vi "GUI_Plasma2_MedJet.vi"() -> ()   [LabVIEW 2013]
uses:
  Shared/GUI_Template/GUI_master/tcp_new_data_event.ctl
  Shared/GUI_Template/GUI_master/tcp new data cluster.ctl
  Control 1.ctl
panel:
  in  "PressureSetPoint.device 1::1":dbl=0.001 caption="Alicat HP Set" min=0.0 max=20.0 format="%_4f"
  in  "PressureSetPoint.device 2::1":dbl=0.001 caption="Alicat LP Set" min=0.0 max=20.0 format="%_4f"
  in  "GUIdevice 1":T1="PL2-PresCtl" caption="PL2-PresCtrl"
  in  "stop":bool
  in  "All Off":bool
  in  "PressureReading.device 1::1":dbl=0.001 caption="Alicat HP Read" min=-10.0 max=20.0 format="%_4f"
  in  "PressureReading.device 2::1":dbl=0.001 caption="Alicat LP Read" min=-10.0 max=20.0 format="%_4f"
  in  "High Valve":bool
  in  "Low Valve":bool
  in  "LN Set Pressure":dbl
  in  "HN Set Pressure":dbl
  out "tcp data event":T2
  out "error IO 2":errorcluster
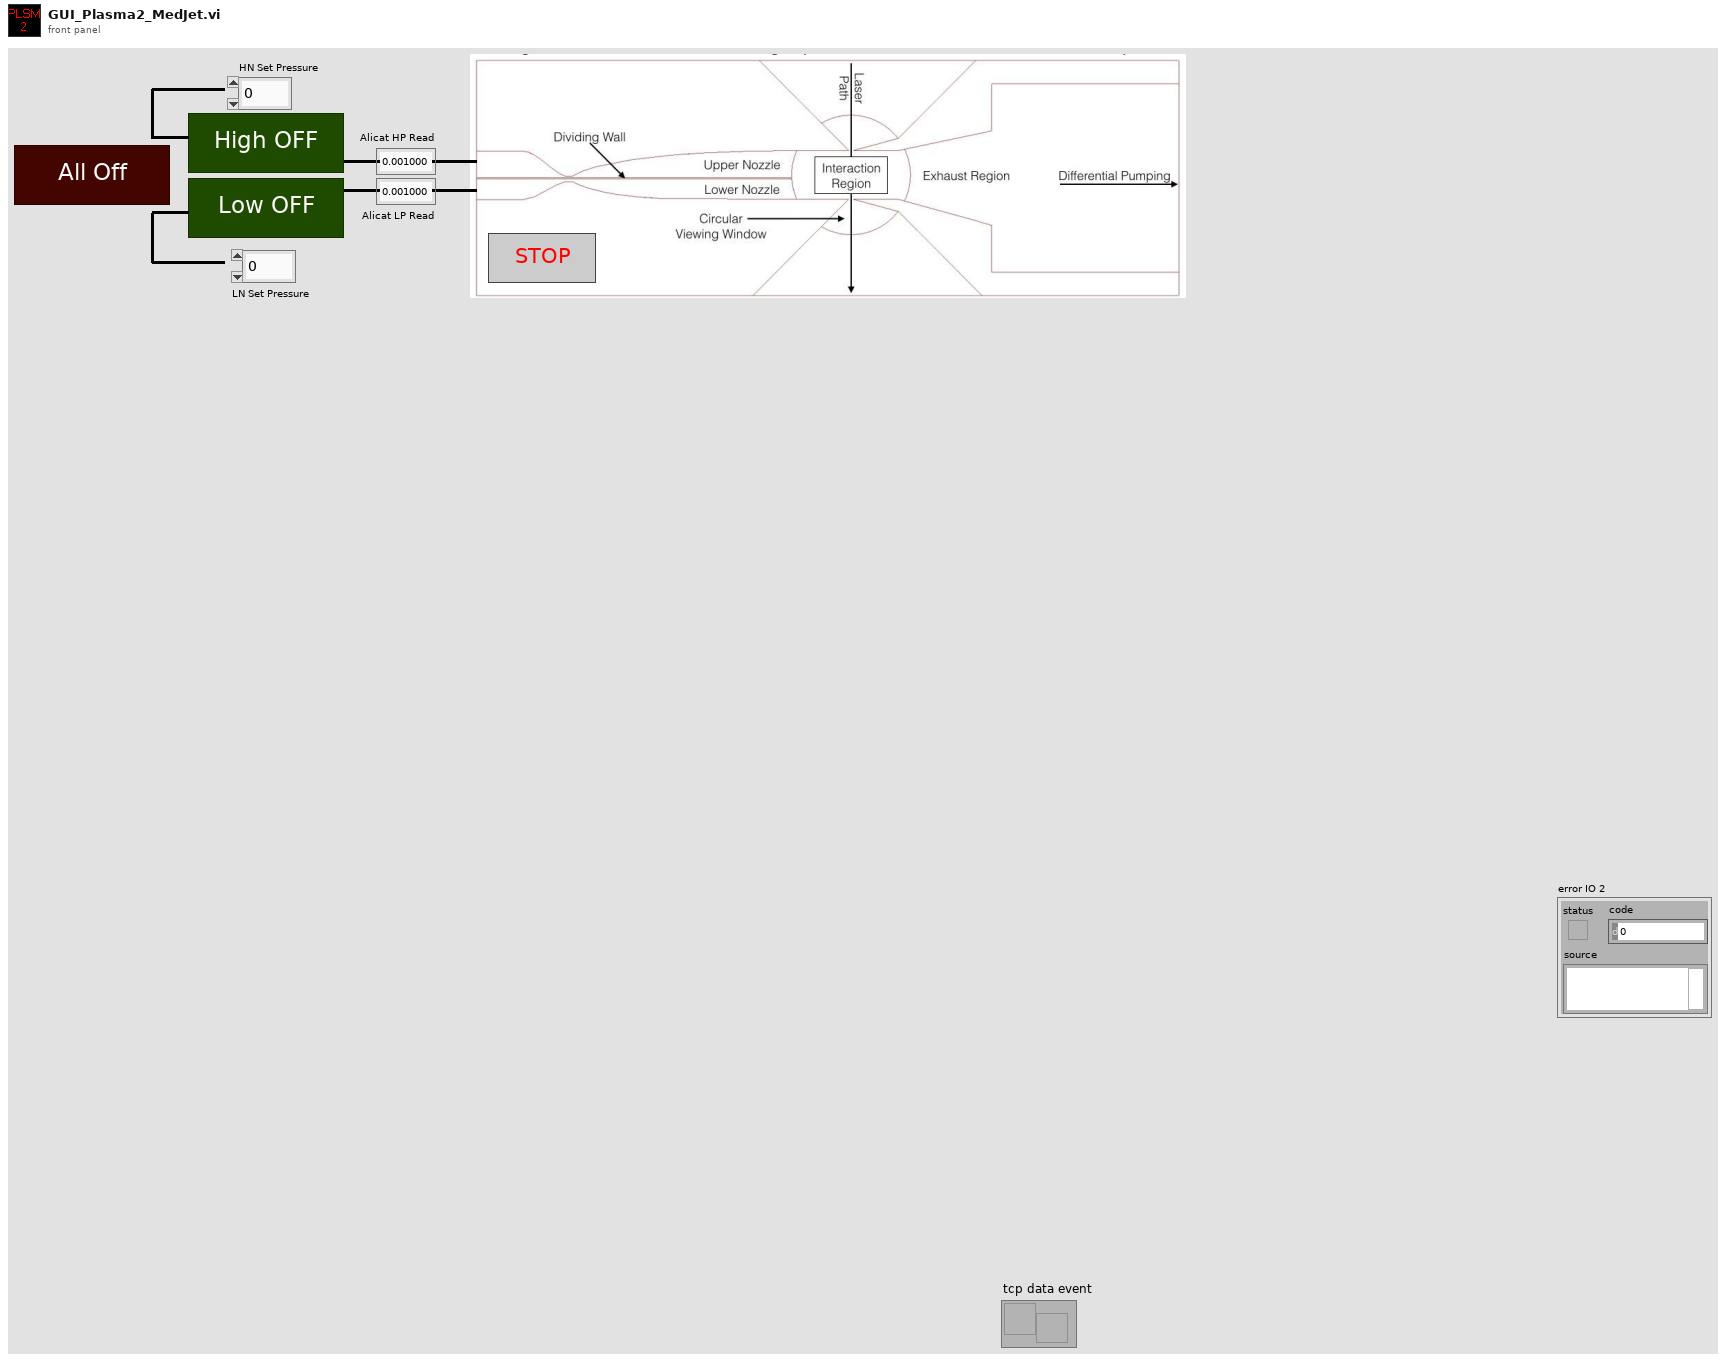
[diagram p1: front panel]
types:
  T1 = typedef "Control 1.ctl" = string
  T2 = typedef "tcp_new_data_event.ctl" = refnum<user-event>
  T3 = typedef "tcp new data cluster.ctl" = cluster{"EventEnum":enum16{"new data", "connection status update"}, "Device name":string}
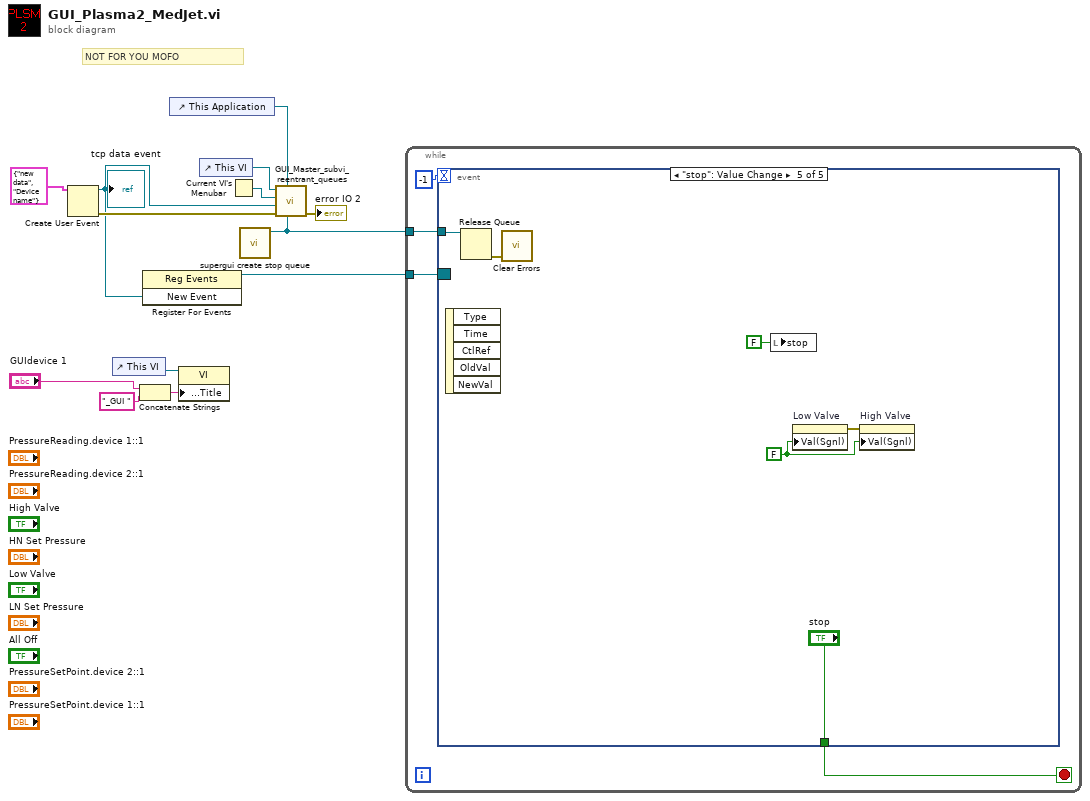
[diagram p0: block diagram]
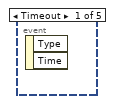
[diagram p2: hidden frame]
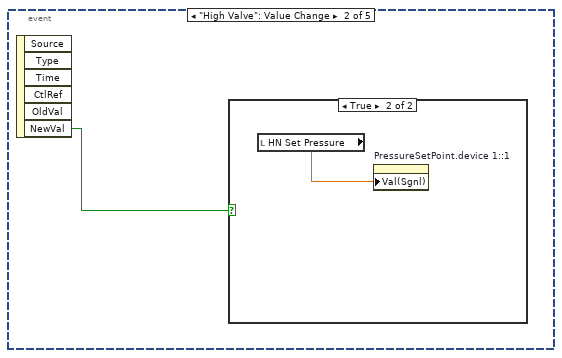
[diagram p3: hidden frame]
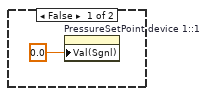
[diagram p4: hidden frame]
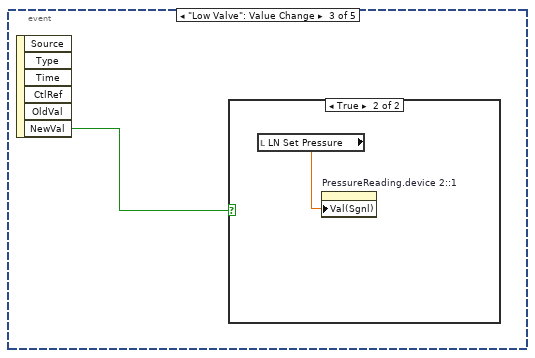
[diagram p5: hidden frame]
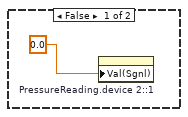
[diagram p6: hidden frame]
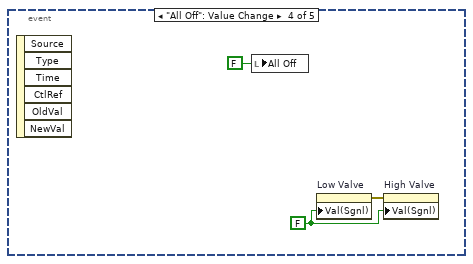
[diagram p7: hidden frame]
diagram:
  # "NOT FOR YOU MOFO"
  n1 = Create User Event(user event datatype=T3 {"EventEnum"=enum."new data", "Device name"="Device name"} ("New Event")) -> (user event=w8:refnum<user-event>, error out=w9:errorcluster)  [unwired: 1 in]
  "tcp data event" <- w8
  n2 = control-ref of="This VI"() -> (w4:refnum<vi>)
  n3 = Concatenate Strings("GUIdevice 1", "_GUI ") -> (w3:string)
  n4 = register-events(w8) -> (reference out=w6:refnum<event-registration>)  [unwired: 2 in, 1 out]
  n5 = control-ref of="This Application"() -> (w7:refnum<vi>)
  n6 = property class="VI"(reference=w4, "Front Panel.Title"=w3) -> ()  [unwired: 1 in, 2 out]
  n7 = control-ref of="This VI"() -> (w12:refnum<vi>)
  n8 = Current VI's Menubar() -> (w11:refnum<k9>)
  n9 = call "supergui create stop queue.vi"() -> ("STOP Queue out"=w5:refnum<queue>)  [unwired: 11 in]
  n10 = call "GUI_Master_subvi_reentrant_queues.vi"("STOP Queue in"=w5, "This Application"=w7, "error in (no error)"=w9, "tcp data event"=w8, "Caller menu reference"=w11, "Caller VI ref"=w12) -> ("error out"=→"error IO 2":errorcluster)  [unwired: 5 in]
  n11 = while {
    tunnel: w6 -> [w16]
    tunnel: w5 -> [w14]
    stop <- w17 stop-if-true
    n12 = event shown="[4] \"stop\": Value Change" {
      selector: w16 -> [_ _ _ _ _]
      dyn-events: _ -> [_ _ _ _ _]
      timeout: -1 -> [_ _ _ _ _]
      tunnel: [_ _ _ _ "stop"] -> w17
      tunnel: w14 -> [_ _ _ _ w27]
      event Timeout {
        n13 = event-data() -> ()  [unwired: 1 in, 2 out]
      }
      event "High Valve": Value Change {
        n14 = event-data() -> ("NewVal"=w18:bool)  [unwired: 1 in, 5 out]
        n15 = case shown="True" w18 {
          frame False {
            n16 = property on="PressureSetPoint.device 1::1" class="DigNum (strict)"("Val(Sgnl)"=0.0 ("HP Set Pressure")) -> ()  [unwired: 2 in, 2 out]
          }
          frame True {
            n17 = local read "HN Set Pressure"() -> (w20:dbl)
            n18 = property on="PressureSetPoint.device 1::1" class="DigNum (strict)"("Val(Sgnl)"=w20) -> ()  [unwired: 2 in, 2 out]
          }
        }
      }
      event "Low Valve": Value Change {
        n19 = event-data() -> ("NewVal"=w21:bool)  [unwired: 1 in, 5 out]
        n20 = case shown="True" w21 {
          frame False {
            n21 = property on="PressureReading.device 2::1" class="DigNum (strict)"("Val(Sgnl)"=0.0 ("HP Set Pressure")) -> ()  [unwired: 2 in, 2 out]
          }
          frame True {
            n22 = local read "LN Set Pressure"() -> (w23:dbl)
            n23 = property on="PressureReading.device 2::1" class="DigNum (strict)"("Val(Sgnl)"=w23) -> ()  [unwired: 2 in, 2 out]
          }
        }
      }
      event "All Off": Value Change {
        w25 = FALSE
        n24 = event-data() -> ()  [unwired: 1 in, 6 out]
        n25 = local write "All Off"(FALSE ("All Off")) -> ()
        n26 = property on="Low Valve" class="Bool (strict)"("Val(Sgnl)"=w25) -> (error out=w24:errorcluster)  [unwired: 2 in, 1 out]
        n27 = property on="High Valve" class="Bool (strict)"(error in=w24, "Val(Sgnl)"=w25) -> ()  [unwired: 1 in, 2 out]
      }
      event "stop": Value Change {
        w30 = FALSE
        n28 = event-data() -> ()  [unwired: 1 in, 5 out]
        n29 = Release Queue(queue=w27) -> (error out=w28:errorcluster)  [unwired: 2 in, 2 out]
        n30 = call <vilib>:"Clear Errors.vi"("error in (no error)"=w28) -> ()  [unwired: 6 in, 1 out]
        n31 = local write "stop"(FALSE ("stop")) -> ()
        n32 = property on="Low Valve" class="Bool (strict)"("Val(Sgnl)"=w30) -> (error out=w29:errorcluster)  [unwired: 2 in, 1 out]
        n33 = property on="High Valve" class="Bool (strict)"(error in=w29, "Val(Sgnl)"=w30) -> ()  [unwired: 1 in, 2 out]
      }
    }
  }
